vi "Geometric Matching RPi Monitor.vi"() -> ()   [LabVIEW 2017]
uses:
  <vilib>/vision/NI_Vision_Development_Module.lvlib
  IMAQCV/IMAQCV.lvlib
  IMAQCV/LVOpenCV.lvlib
panel:
  out "Process Time (ms)":dbl format="%.2f"
  out "picture":picture
  out "Template":T1(plugin-control)
  in  "Stop":bool
  out "Number of Matches Found":i32
  in  "Number of Matches":i32=4
  in  "Minimum Score":sgl=800.0
  out "Results":string[][](table)
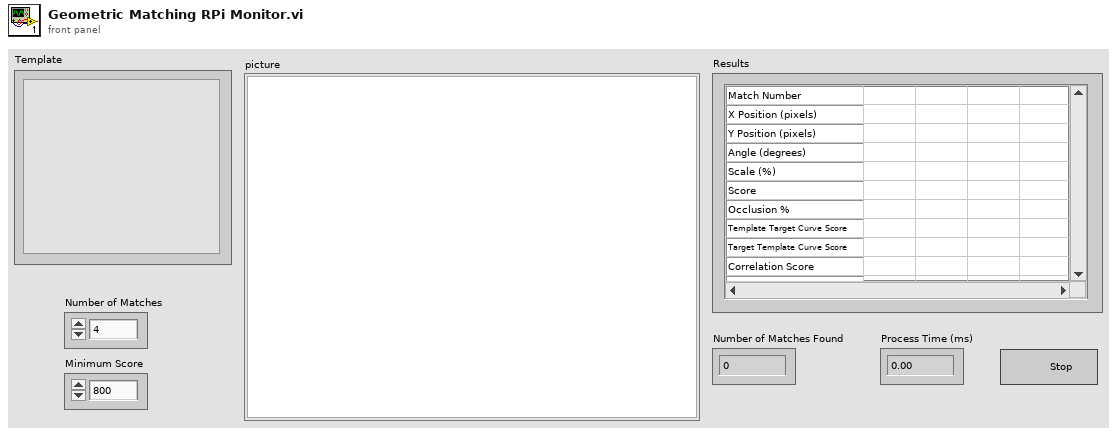
[diagram p1: front panel]
types:
  T1 = typedef "IMAQ Image.ctl" = refnum<image>
  T2 = typedef "Image Type" = u32
  T3 = typedef "IMAQCV.lvlib/IMAQCV Image.ctl" = refnum<vi>
  T4 = cluster{"Rotation":bool, "Scale":bool, "Occlusion":bool, "Reserved":bool, "Reserved":bool, "Reserved":bool}
  T5 = typedef "IMAQ GM Match Report.ctl" = cluster{"Position":cluster{"x":sgl, "y":sgl}, "Angle":sgl, "Scale":sgl, "Score":sgl, "Bounding Box":cluster{"x":sgl, "y":sgl}[], "Contrast Reversed":bool, "Occlusion %":sgl, "Template Target Curve Score":sgl, "Target Template Curve Score":sgl, "Correlation Score":sgl}
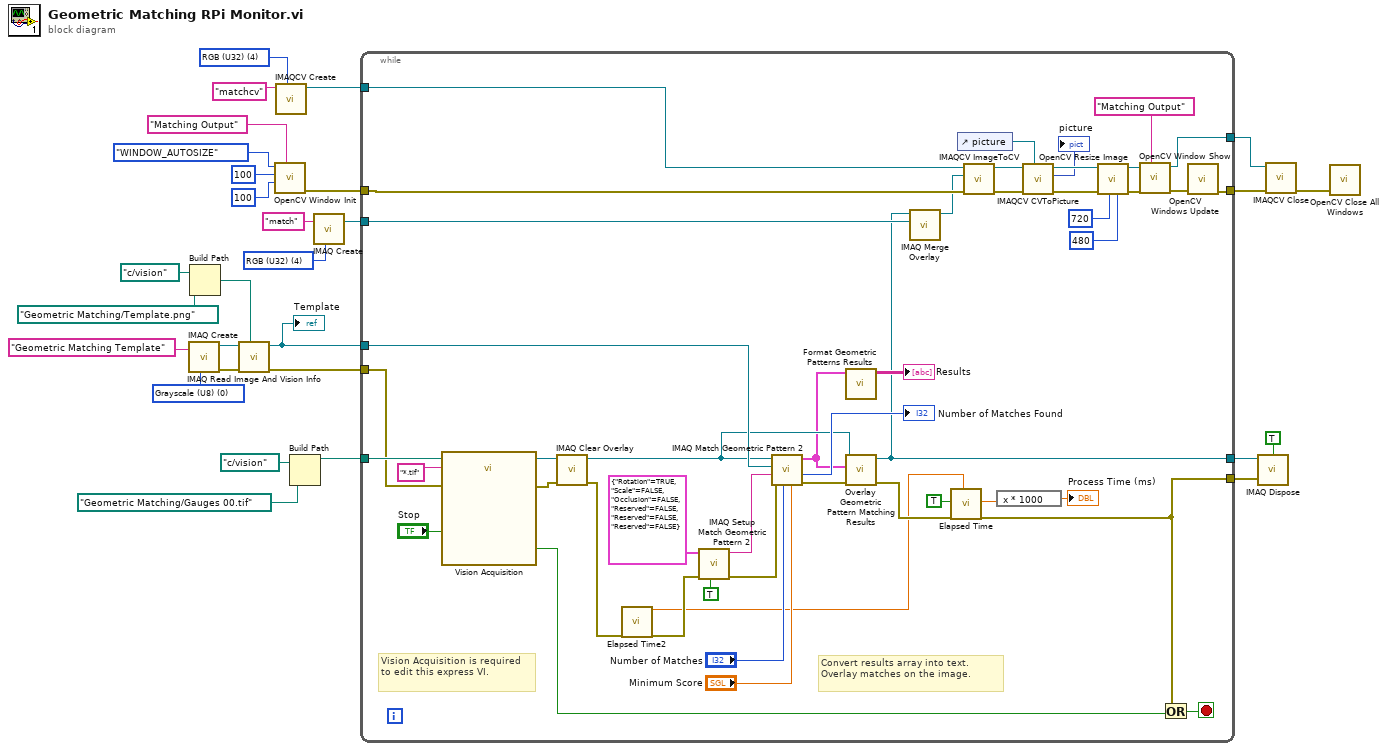
[diagram p0: block diagram]
diagram:
  w11 = T2 4 items=["Grayscale (U8)", "Grayscale (I16)", "Grayscale (SGL)", "Complex (CSG)", "RGB (U32)", "HSL (U32)", "RGB (U64)", "Grayscale (U16)"] ("Image Type")
  w13 = T2 4 items=["Grayscale (U8)", "Grayscale (I16)", "Grayscale (SGL)", "Complex (CSG)", "RGB (U32)", "HSL (U32)", "RGB (U64)", "Grayscale (U16)"] ("Image Type")
  w22 = T2 0 items=["Grayscale (U8)", "Grayscale (I16)", "Grayscale (SGL)", "Complex (CSG)", "RGB (U32)", "HSL (U32)", "RGB (U64)"] ("Image Type")
  n1 = call "IMAQ Create"("Image Name"="Geometric Matching Template", "Image Type"=w22) -> ("New Image"=w23:T1, "error out"=w24:errorcluster)  [unwired: 2 in, 1 out]
  n2 = Build Path(base path=path "c:/vision", name or relative path=path "Geometric Matching/Template.png") -> (appended path=w26:path)
  n3 = call "IMAQ Read Image And Vision Info"("File Path"=w26, "error in (no error)"=w24, "Image"=w23) -> ("error out"=w18:errorcluster, "Image Out"=w20:T1)  [unwired: 1 in, 6 out]
  "Template" <- w20
  n4 = call "OpenCV Window Init.vi"("window name"="Matching Output", "y"=u32 100, "x"=u32 100, "mode"=enum8{"WINDOW_AUTOSIZE", "WINDOW_FULLSCREEN"}."WINDOW_AUTOSIZE") -> ("error out"=w9:errorcluster)  [unwired: 7 in]
  n5 = call "IMAQCV Create.vi"("Image Type"=w13, "Image Name"="matchcv") -> ("Image Out"=w16:T3)  [unwired: 8 in, 1 out]
  n6 = Build Path(base path=path "c:/vision", name or relative path=path "Geometric Matching/Gauges 00.tif") -> (appended path=w28:path)
  n7 = call "IMAQ Create"("Image Name"="match", "Image Type"=w11) -> ("New Image"=w10:T1)  [unwired: 2 in, 2 out]
  n8 = while {
    tunnel: w28 -> [w75]
    tunnel: [w36] -> w27
    tunnel: w20 -> [w61]
    tunnel: [w52] -> w19
    tunnel: w18 -> [w60]
    tunnel: w9 -> [w55]
    tunnel: w16 -> [w56]
    tunnel: [w54] -> w15
    tunnel: w10 -> [w53]
    tunnel: [w44] -> w3
    stop <- w72 stop-if-true
    # "Vision Acquisition is required to edit this express VI."
    # "Convert results array into text.\nOverlay matches on the image."
    n9 = call "Vision Acquisition"("Image Path"=w75, "Image File Type (All Types)"="*.tif", "Stop (F)"="Stop", "error in"=w60) -> ("Image Out"=w71:T1, "Stopped"=w73:bool, "error out"=w74:errorcluster)  [unwired: 21 in]
    n10 = call "IMAQ Clear Overlay"("error in (no error)"=w74, "Image"=w71) -> ("error out"=w35:errorcluster, "Image Out"=w59:T1)  [unwired: 1 in, 7 out]
    n11 = call "Elapsed Time2"("error in (no error)"=w35) -> ("Present (s)"=w33:dbl, "error out"=w34:errorcluster)  [unwired: 11 in, 6 out]
    n12 = call "IMAQ Setup Match Geometric Pattern 2"("Use Learn Curve Parameters"=TRUE, "error in (no error)"=w34, "Match Mode"=T4 {"Rotation"=TRUE, "Scale"=FALSE, "Occlusion"=FALSE, "Reserved"=FALSE, "Reserved"=FALSE, "Reserved"=FALSE}) -> ("error out"=w68:errorcluster, "Match Geometric Pattern 2 Setup Data"=w66:string)  [unwired: 3 in, 4 out]
    n13 = call "IMAQ Match Geometric Pattern 2"("Minimum Match Score"="Minimum Score", "Number of Matches Requested"="Number of Matches", "error in (no error)"=w68, "Match Geometric Pattern 2 Setup Data"=w66, "Template Image"=w61, "Image"=w59) -> ("error out"=w63:errorcluster, "Number of Matches"=→"Number of Matches Found":i32, "Matches (pixel)"=w58:T5[])  [unwired: 1 in, 2 out]
    n14 = call "Format Geometric Patterns Results.vi"("Matches"=w58) -> ("Text Results"=→"Results":string[][])  [unwired: 9 in, 1 out]
    n15 = call "Overlay Geometric Pattern Matching Results.vi"("error in"=w63, "Matches"=w58, "Image"=w59) -> ("error out"=w37:errorcluster, "Image Out"=w52:T1)  [unwired: 7 in]
    n16 = call "IMAQ Merge Overlay"("Image Dst"=w53, "Image Src"=w52) -> ("Image Dst Out"=w49:T1)  [unwired: 8 in, 1 out]
    n17 = call "Elapsed Time"("Reset"=TRUE, "error in (no error)"=w37, "Set Start Time (s)"=w33) -> ("Elapsed Time (s)"=w31:dbl, "error out"=w36:errorcluster)  [unwired: 9 in, 6 out]
    n18 = control-ref of="picture"() -> (w38:refnum<vi>)
    n19 = call "IMAQCV ImageToCV.vi"("error in (no error)"=w55, "Variant In"=w49, "CV in"=w56) -> ("error out"=w43:errorcluster, "CV out"=w42:T3)  [unwired: 7 in]
    n20 = expression code="x * 1000"(w31) -> (→"Process Time (ms)":dbl)
    n21 = call "IMAQCV CVToPicture.vi"("picture ref"=w38, "error in (no error)"=w43, "image"=w42) -> ("error out"=w40:errorcluster, "picture"=→"picture":picture, "image out"=w41:T3)  [unwired: 6 in]
    n22 = call "OpenCV Resize Image.vi"("height"=u32 480, "width"=u32 720, "error in (no error)"=w40, "image in"=w41) -> ("error out"=w47:errorcluster, "image out"=w48:T3)  [unwired: 6 in]
    n23 = call "OpenCV Window Show.vi"("window name"="Matching Output", "error in (no error)"=w47, "image in"=w48) -> ("error out"=w50:errorcluster, "image out"=w44:T3)  [unwired: 7 in]
    n24 = Or(x=w36, y=w73) -> (x .or. y?=w72:bool)
    n25 = call "OpenCV Windows Update.vi"("error in (no error)"=w50) -> ("error out"=w54:errorcluster)  [unwired: 9 in, 1 out]
  }
  n26 = call "IMAQ Dispose"("All Images? (No)"=TRUE, "Image"=w19, "error in (no error)"=w27) -> ()  [unwired: 4 out]
  n27 = call "IMAQCV Close.vi"("error in (no error)"=w15, "Image"=w3) -> ("error out"=w2:errorcluster)  [unwired: 9 in]
  n28 = call "OpenCV Close All Windows.vi"("error in (no error)"=w2) -> ()  [unwired: 10 in, 1 out]
